vi "Init Runtime.vi"(8 "error in (no error)":errorcluster, 11 "csv-formatter Config in":refnum<class "csv-formatter Config.lvclass">) -> (0 "error out":errorcluster, 2 "Formatter.lvclass":refnum<class "Formatter.lvclass">, 3 "csv-formatter Config out":refnum<class "csv-formatter Config.lvclass">)   [LabVIEW 2015, in "csv-formatter Config.lvclass"]
uses:
  csv-formatter Config.lvclass
  Base Class/Execution/Formatter.lvclass
  Execution/csv-formatter.lvclass
  csv-formatter Config.lvclass/csv-formatter Config.ctl
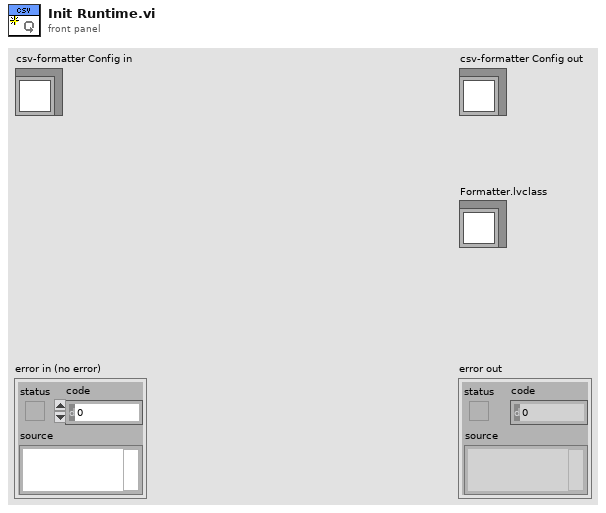
[diagram p1: front panel]
types:
  T1 = typedef "Result Config.ctl" = string[]
  T2 = typedef "Report Header Config.ctl" = string[][]
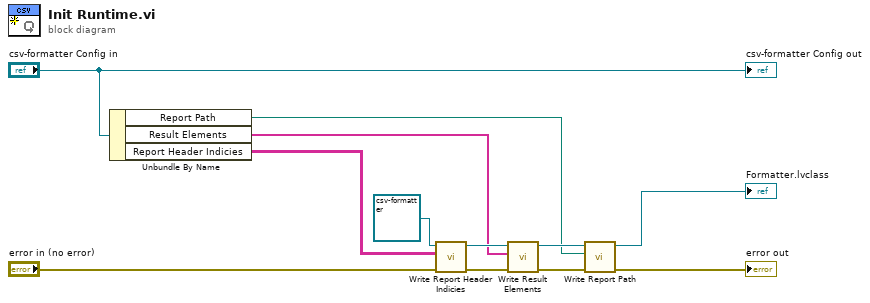
[diagram p0: block diagram]
diagram:
  n1 = Unbundle By Name("csv-formatter Config in") -> ("Report Path"=w7:path, "Result Elements"=w8:T1, "Report Header Indicies"=w9:T2)
  n2 = call-dynamic "Write Report Header Indicies.vi"("error in (no error)"="error in (no error)", "Report Header Indicies"=w9, "csv-formatter in"=refnum<class "csv-formatter.lvclass"> refnum ("csv-formatter.lvclass")) -> ("error out"=w5:errorcluster, "csv-formatter out"=w12:refnum<class "csv-formatter.lvclass">)  [unwired: 7 in]
  n3 = call-dynamic "Write Result Elements.vi"("error in (no error)"=w5, "Result Elements"=w8, "csv-formatter in"=w12) -> ("error out"=w4:errorcluster, "csv-formatter out"=w10:refnum<class "csv-formatter.lvclass">)  [unwired: 7 in]
  n4 = call-dynamic "Write Report Path.vi"("error in (no error)"=w4, "Report Path"=w7, "csv-formatter in"=w10) -> ("error out"=→"error out":errorcluster, "csv-formatter out"=→"Formatter.lvclass":refnum<class "csv-formatter.lvclass">)  [unwired: 7 in]
  "csv-formatter Config out" <- "csv-formatter Config in"
